vi "ChannelAutomatorR_Whole.vi"() -> ()   [LabVIEW 2024]
uses:
  E:/CodeProjects/DEMPbot/ChannelAutomatorR2/PumpAdapter.exe
  PumpAdapter.exe
  <vilib>/Analysis/baseanly.llb/Mean (DBL).vi
  <vilib>/DAQmx/write.llb/DAQmx Write (Analog DBL 1Chan 1Samp).vi
  <vilib>/DAQmx/create/channels.llb/DAQmx Create Channel (AO-Voltage-Basic).vi
  <vilib>/DAQmx/create/channels.llb/DAQmx Create Channel (AI-Voltage-Basic).vi
  <vilib>/DAQmx/miscellaneous.llb/DAQmx Fill In Error Info.vi
  <vilib>/DAQmx/configure/timing.llb/DAQmx Timing (Sample Clock).vi
  <vilib>/Analysis/NI_AALBase.lvlib
panel:
  in  "Run Experiment":bool
  out "Pull":string
  out "LastTDMS":refnum<k34>
  out "ChannelHistory":refnum<k24>
  out "Array":dbl[](array[numeric])
  out "Stats":string[][](table)
  out "History":cluster{dbl[], dbl[]}[](graph)
  out "Pump":refnum<k24>
  out "First Time":i64
  out "LastPoint":i64
  out "biasChannel":refnum<k21>
  out "HistoryArray":T1(array[cluster])
  out "MeasureMode":enum32{"RT Monitor", "IV Monitor"}(ring)
  out "error out 4":errorcluster
  out "fileCreateTime":timestamp
  out "error out 2":errorcluster
  in  "Tab Control 2":T2(tab)
  out "Channel 4":waveform(dbl)[](graph)
  out "Channel 3":waveform(dbl)[](graph)
  out "Channel 2":waveform(dbl)[](graph)
  out "Channel 1":waveform(dbl)[](graph)
  out "XY Graph":cluster{"Y":dbl[], "Y":dbl[]}[](graph)
  out "XY Graph 2":cluster{"Y":dbl[], "Y":dbl[]}[](graph)
  out "XY Graph 3":cluster{"Y":dbl[], "Y":dbl[]}[](graph)
  out "XY Graph 4":cluster{"Y":dbl[], "Y":dbl[]}[](graph)
  in  "Experiment":string[][](table)=[["Air", "", "Air", "0", "", "", "", "", "1", "200", "5", "IV Curve", "", ""], ["Air", "", "Air", "0", "", "", "", "", "5", "200", "5", "", "", ""], ["", "pushonly", "Water", "1800", "200", "", "", "", "", "", "", "", "", ""], ["TimEtch", "pushonly", "Waste", "500", "200", "", "", "", "", "50", "", "RT Start", "", ""], ["TE_Rinse", "", "Water", "3000", "200", "", "", "", "", "", "", " ", "", ""], ["", "", "", "0", "", "", "", "", "", "50", "", "RT End", "", ""], ["TE_Rinse", "", " ", "0", "", "", "", "", "5", "200", "5", "IV Curve", "", ""], ["MPA", "pullmore", "MPA", "300", "200", "", "1000", "", "", "", "", " ", "", ""], ["", "", "Air", "100", "200", "", "", "", "", "50", "", "RT Start", "", ""], ["MPA", "", "Water", "1600", "100", "", "", "", "", "", "", "", "", ""], ["", "", "MPA", "0", "", "", "", "", "0", "50", "", "RT End", "", ""], ["", "", "MPA", "0", "", "", "", "", "360", "100", "", "Burst", "60", "1"], ["MPA Rinse", "", "Water", "3000", "100", "", "", "", "60", "100", "", "", "", ""], ["MPA Rinse", "", "MPARinse", "0", "", "", "", "", "5", "100", "5", "IV Curve", "", ""], ["", "", "", "", "", "", "", "", "", "", "", "", "", ""], ["", "", "", "", "", "", "", "", "", "", "", "", "", ""], ["", "", "", "", "", "", "", "", "", "", "", "", "", ""], ["", "", "", "", "", "", "", "", "", "", "", "", "", ""], ["", "", "", "", "", "", "", "", "", "", "", "", "", ""], ["", "", "", "", "", "", "", "", "", "", "", "", "", ""], ["", "", "", "", "", "", "", "", "", "", "", "", "", ""], ["", "", "", "", "", "", "", "", "", "", "", "", "", ""]]
  out "output path":path
  out "FilenameValid":bool
  out "ParameterNames":string[](array[string])=["Wafer", "Notes", "Experiment Name", "Buffer", "Bias Voltage", "Reference Electrode", "Chip", "Analyte"]
  out "ParameterValues":string[](array[string])
  out "RT Monitoring 2":bool
  out "error out":errorcluster
  out "StopProgram":bool
  out "FileOpen":bool
  out "tdms file out":refnum<k34>
  in  "Tab Control":enum32{"Data View", "Automation", "Settings"}(tab)
  in  "Current Step":dbl
  in  "TraceTime":dbl=30.0
  in  "IV Monitoring":bool
  in  "RT Monitoring":bool
  out "Recording":bool
  in  "Record":bool
  in  "Reference Voltage (mV)":string="100"
  in  "Bias Voltage (mV)":string="100"
  in  "Experiment Name":string="asdf"
  in  "Wafer, Chip":string="asdf,a"
  in  "Notes":string
  in  "Buffer":string="asdf"
  in  "Analyte":string
  in  "DB48":bool
  in  "DB37":bool
  in  "Device Banks":bool
  in  "DB26":bool
  in  "Channels":string="N2,N6,E2,E6,S2,S6,W2,W6"
  out "Warnings":string="Wrong number of Channel Names!"
  out "Monitoring":bool
  out "frequency":dbl=20.0
  out "Running Experiment":bool
  in  "LoadPort":bool
  in  "Port To Clean":string="MPA"
  in  "CleanPort":bool
  in  "SyringeVolume":dbl=1000.0
  in  "CleanAll":bool
  in  "MPA Load":bool
  in  "PrimeWater":bool
  in  "TimeEtch Back":bool
  in  "ClearInput":bool
  in  "Clear Waste":bool
  in  "Dead Volume":dbl=3000.0
  in  "DataDirectory":path=path "C:/DempBot_Data"
  in  "Sampling Rate:":dbl=5000.0
  in  "Recorded Channels":i32=8
  in  "No. of Samples / Loop":i64=1000
  in  "Gain (V/nA)":dbl=0.45
  in  "Bias channel":tag="Dev1/ao0"
  in  "anayteNames":string[](array[string])=["Water", "TimEtch", "Air", "Dispense", "Waste", "MPA", "Biotin", "SA"]
  in  "Channels 2":tag[](array[tag])=["Dev1/ai0", "Dev1/ai1", "Dev1/ai2", "Dev1/ai3", "Dev1/ai4", "Dev1/ai5", "Dev1/ai6", "Dev1/ai7"]
  in  "MaxSyringSpeed":dbl=1000.0
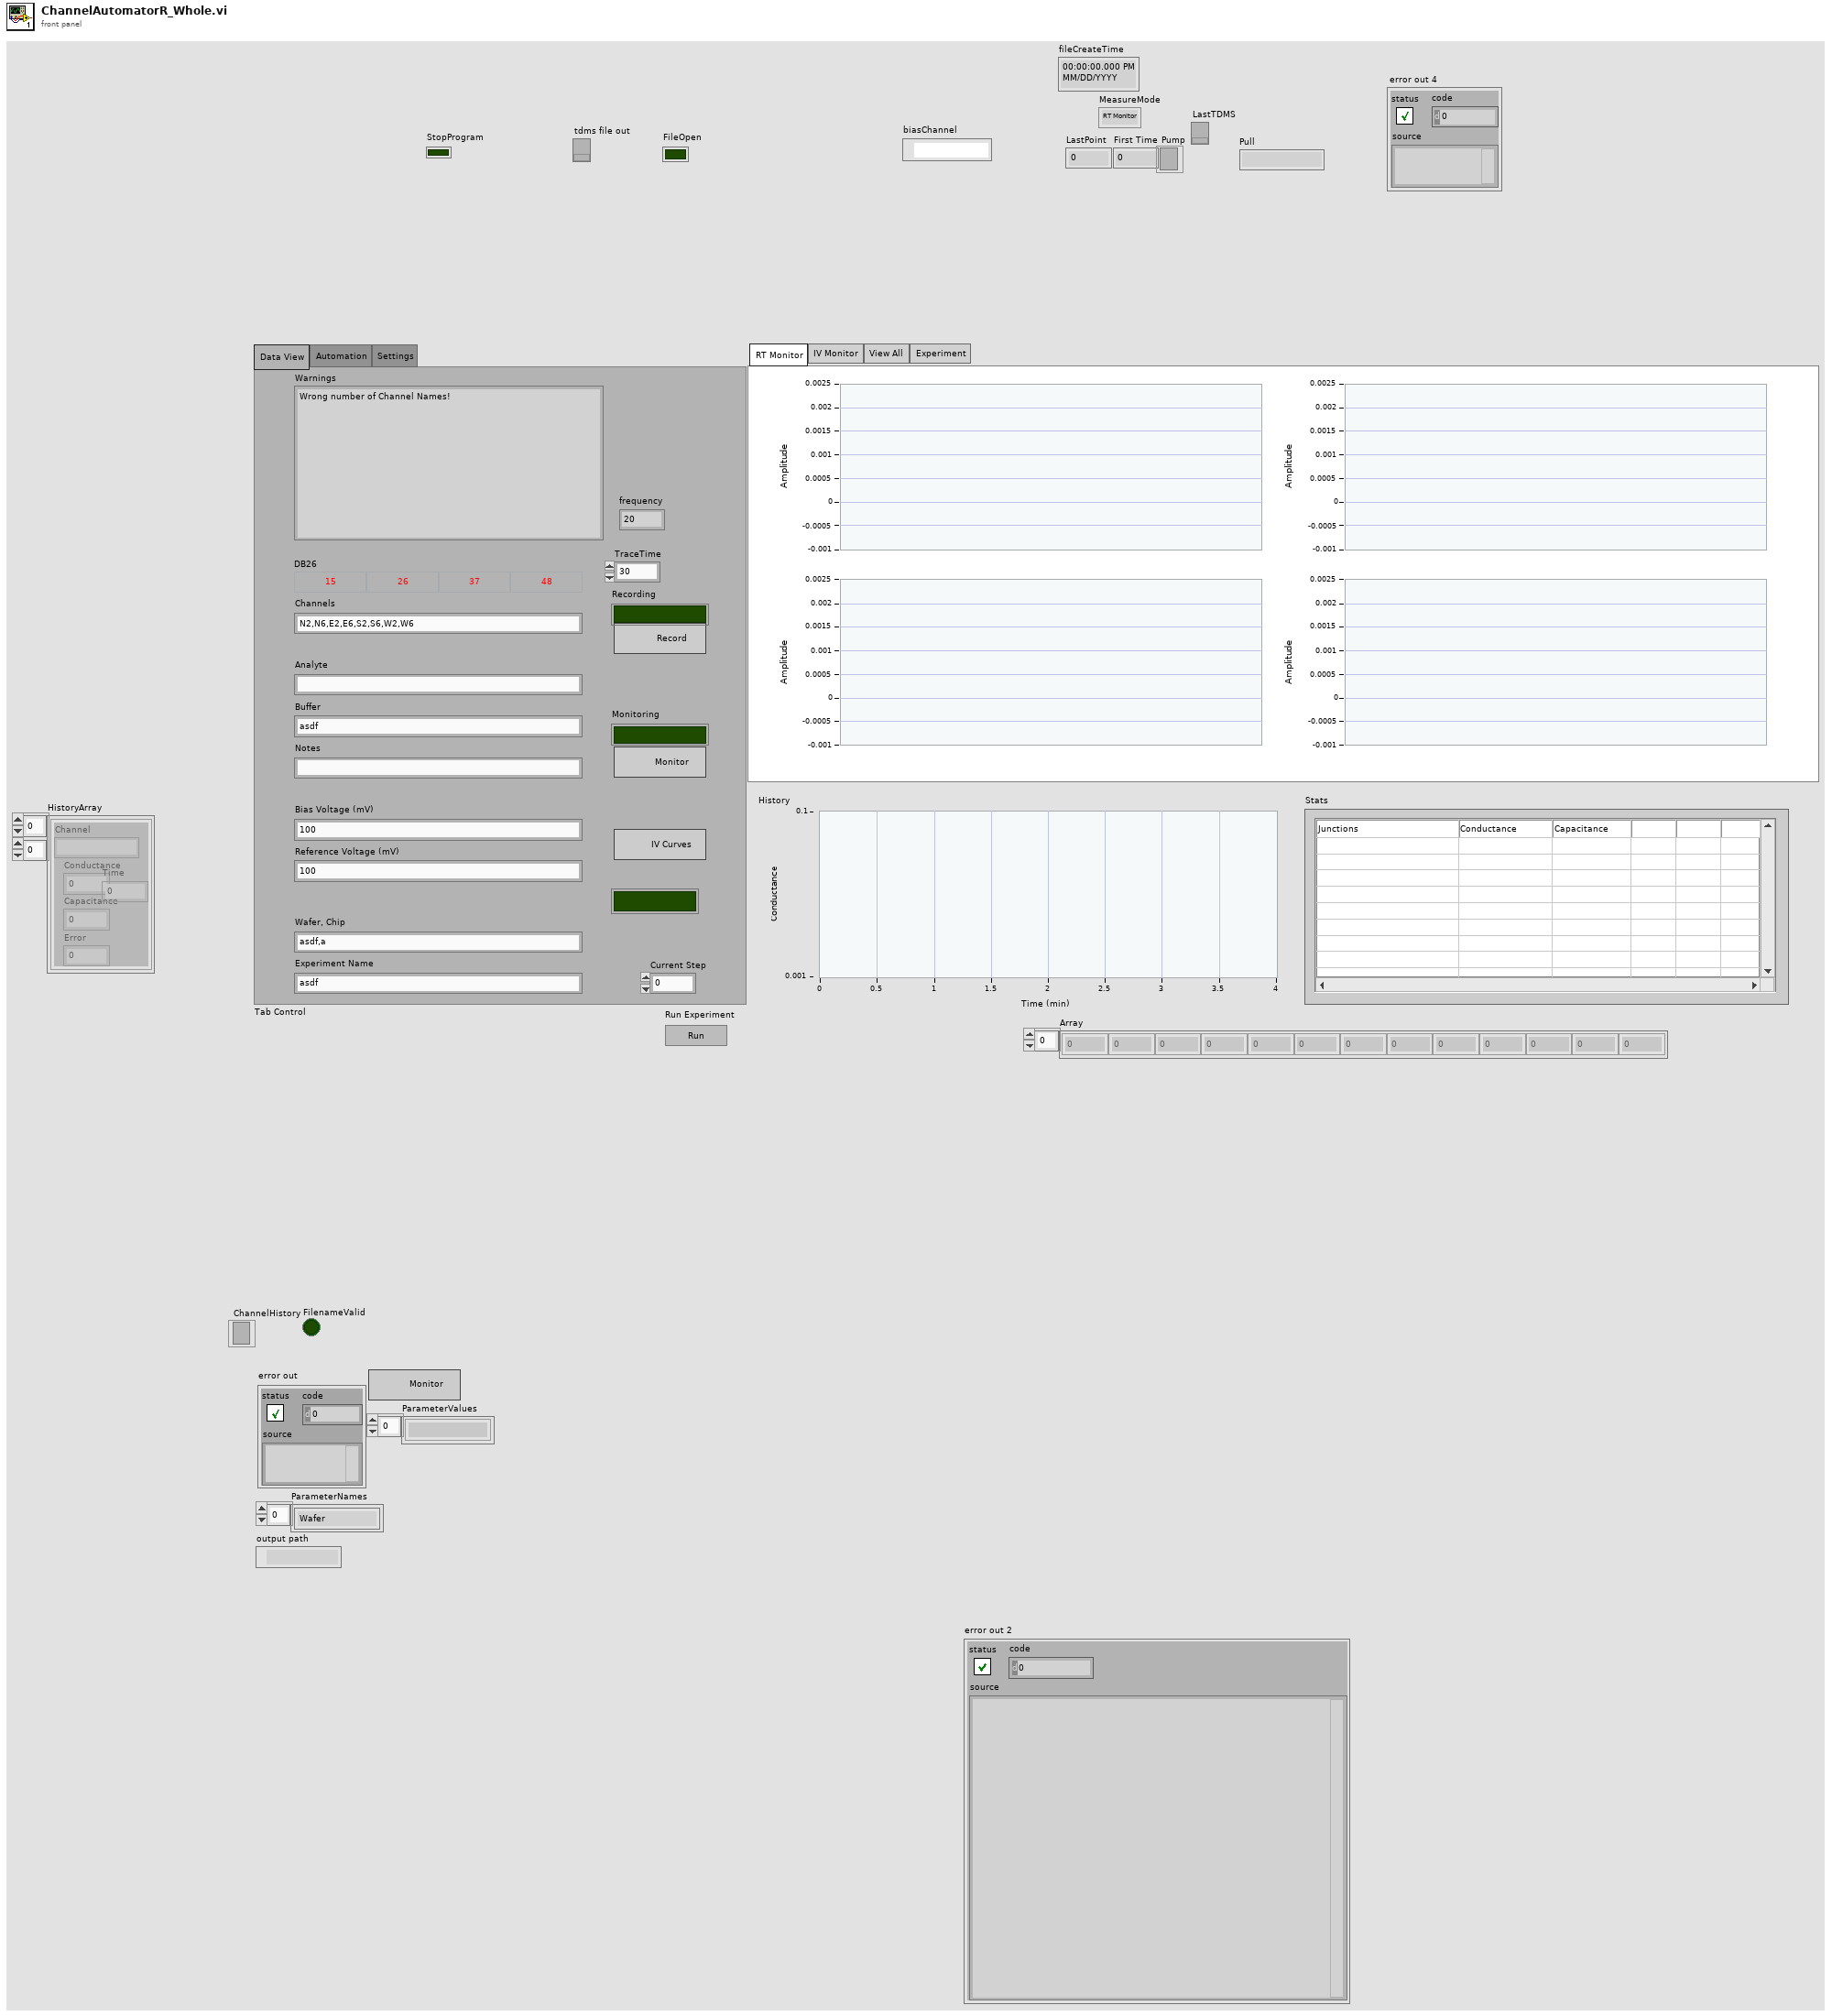
[diagram p1: front panel]
types:
  T1 = cluster{"Channel":string, "Conductance":dbl, "Capacitance":dbl, "Error":dbl, "Time":dbl}[][]
  T2 = enum32{"RT Monitor", "IV Monitor", "View All", "Experiment"}
  T3 = cluster{"Channel":string, "Conductance":dbl, "Capacitance":dbl, "Error":dbl}[][]
  T4 = typedef "MessageQueues.ctl" = cluster{"DelayTime":refnum<queue>, "DownSampled":refnum<queue>, "UserCommands":refnum<queue>, "InternalCommands":refnum<queue>, "CommandType":cluster{"Command":string}, "CommandAndPayload":cluster{"command":string, "machine":string, "payload":string}, "client handle out":T5, "PostData":string, "GetCommand":string, "Ack":string, "VoltageProgram":refnum<queue>, "ExperimentCommands":refnum<queue>, "DisplayCurrents":refnum<queue>, "MonitorCurrents":refnum<queue>, "FilePile":refnum<queue>}
  T5 = typedef "LabVIEWHTTPClient.lvlib/ClientHandle.ctl" = refnum<k1>
  T6 = enum16{"open", "open or create", "create or replace", "create", "open (read-only)"}
  T7 = cluster{"Waveforms":waveform(dbl)[], "file":refnum<k34>}[]
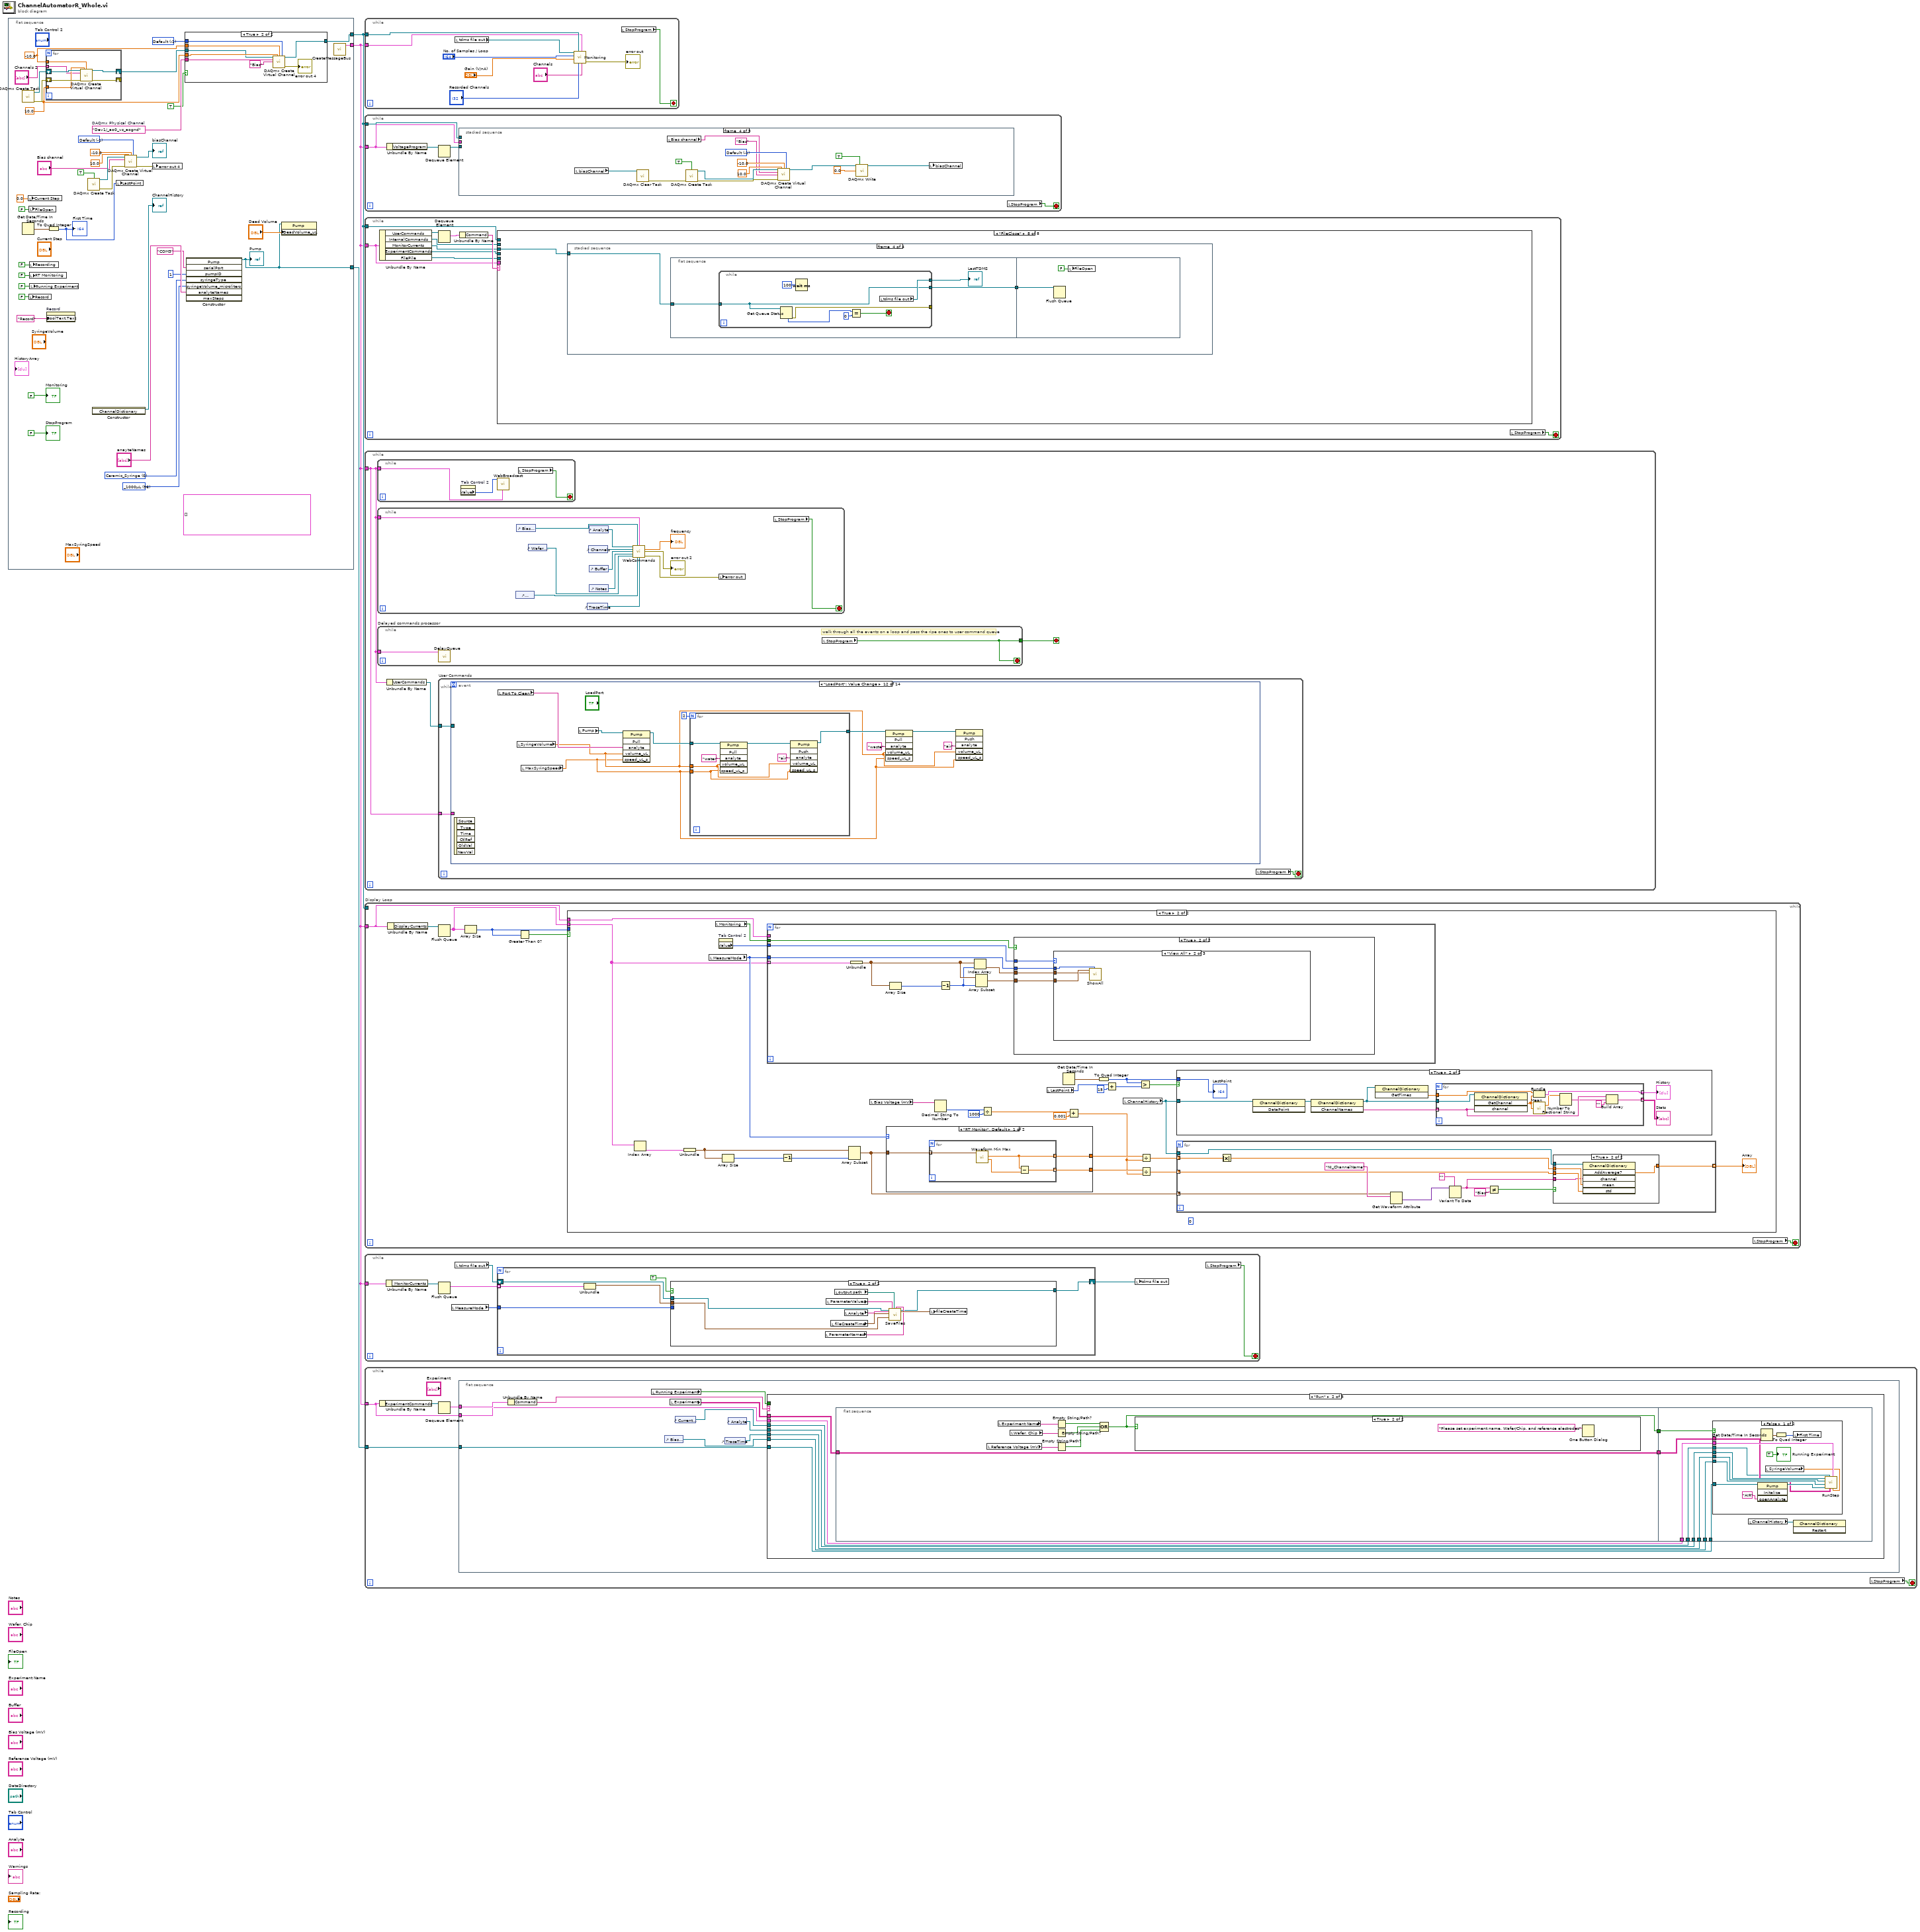
[diagram p0: block diagram]
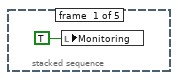
[diagram p7: hidden frame]
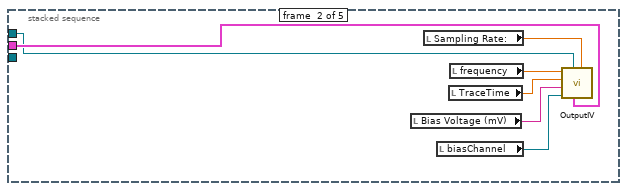
[diagram p8: hidden frame]
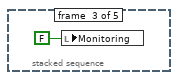
[diagram p9: hidden frame]
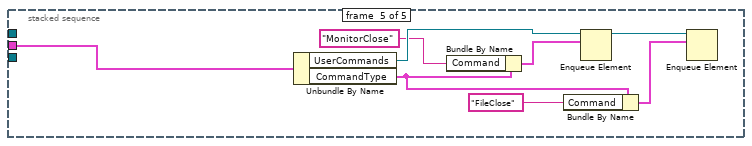
[diagram p10: hidden frame]
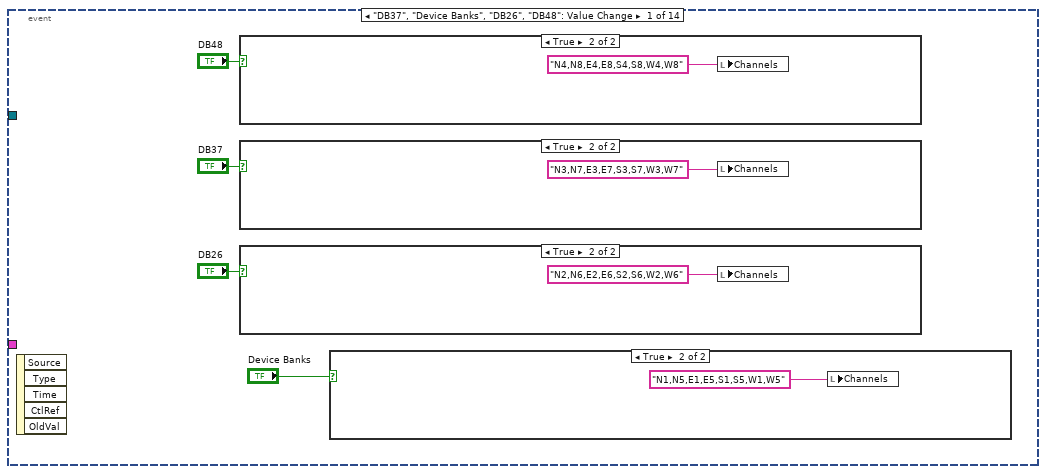
[diagram p11: hidden frame]
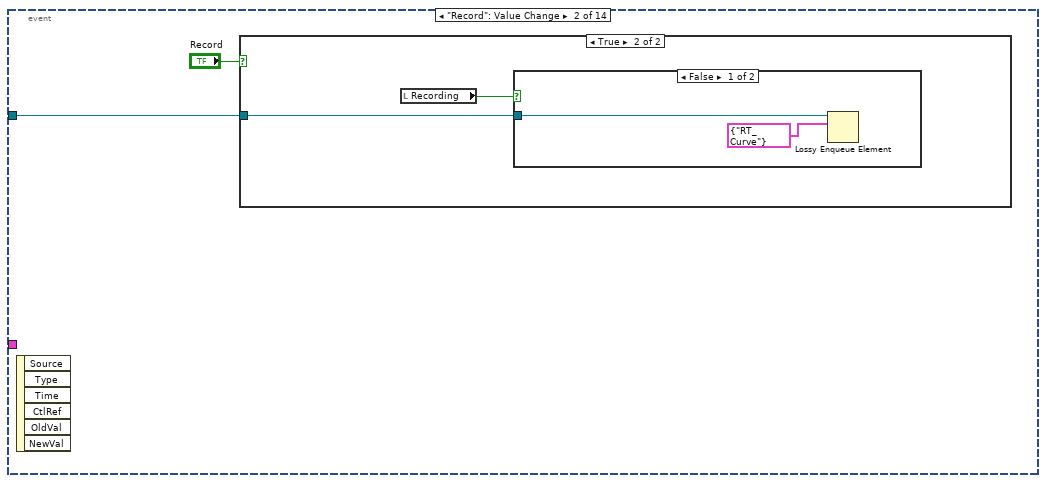
[diagram p16: hidden frame]
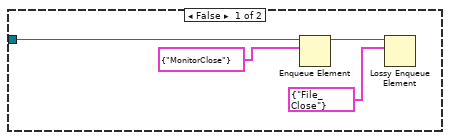
[diagram p17: hidden frame]
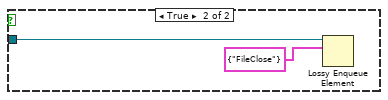
[diagram p18: hidden frame]
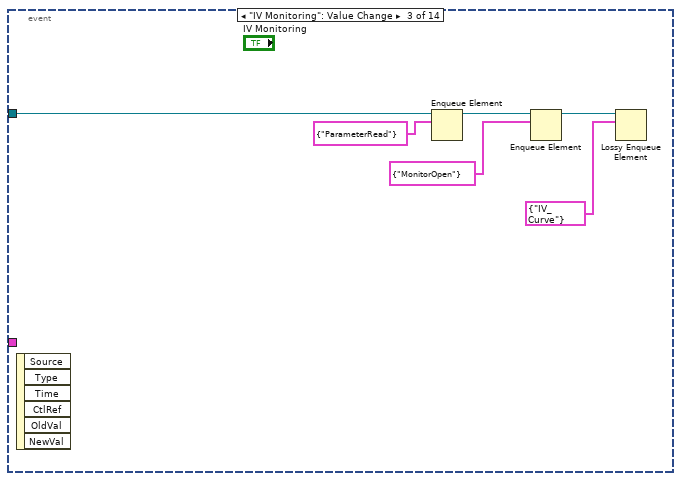
[diagram p19: hidden frame]
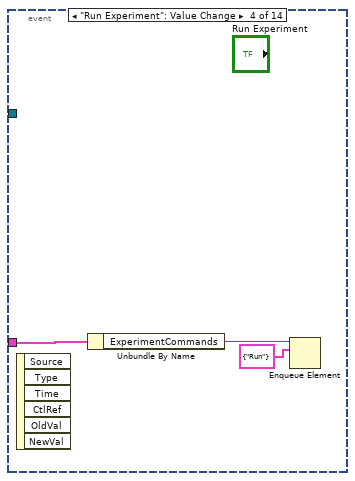
[diagram p20: hidden frame]
diagram:
  n1 = flat-sequence {
    tunnel: [w33] -> w2
    tunnel: [w28] -> w1
    tunnel: [w11] -> w3
    frame #0 {
      w8 = 0 items=["Ceramic_Syringe"=0, "Glass_Syringe"=2000, "Ceramic_Syringe_W_Wash"=2300, "Large_Glass_Syringe"=4000] ("syringeType")
      w9 = 96 items=["_250uL"=90, "_1250uL"=91, "_5000µL"=92, "_50µL"=93, "_100µL"=94, "_500µL"=95, "_1000µL"=96, "_2500µL"=97, "_12500µL"=98] ("syringeVolume_microliters")
      w23 = -1 items=["Default"=-1, "RSE"=10083, "Differential"=10106, "Pseudodifferential"=12529] ("output terminal configuration")
      (unwired) T3 []
      w31 = -1 items=["Default"=-1, "RSE"=10083, "NRSE"=10078, "Differential"=10106, "Pseudodifferential"=12529] ("input terminal configuration")
      w34 = tag "Dev1/_ao0_vs_aognd"  # DAQmx Physical Channel
      w30 = -10.0 ("minimum value")
      w29 = 10.0 ("maximum value")
      n2 = call <vilib>:"DAQmx Create Task.vi"() -> ("task out"=w42:refnum<k21>, "error out"=w41:errorcluster)  [unwired: 14 in]
      n3 = Get Date/Time In Seconds() -> (seconds since 1Jan1904=w13:timestamp)
      n4 = local write "Current Step"(0.0 ("Current Step")) -> ()
      n5 = local write "FileOpen"(FALSE ("FileOpen")) -> ()
      n6 = local write "Record"(FALSE ("Record")) -> ()
      n7 = local write "Recording"(FALSE ("Recording")) -> ()
      n8 = local write "RT Monitoring"(FALSE ("RT Monitoring")) -> ()
      n9 = local write "Running Experiment"(FALSE ("Running Experiment")) -> ()
      n10 = for {
        tunnel: w30 -> [w54]
        tunnel: w29 -> [w53]
        shift-right: [w58] -> w17
        shift-left: w42 -> [w56]
        shift-right: [w57] -> _
        shift-left: w41 -> [w55]
        tunnel: "Channels 2" -> [w52] mode=indexing
        n11 = call-poly <vilib>:"DAQmx Create Virtual Channel.vi"("task in"=w56, "maximum value"=w53, "minimum value"=w54, "physical channels"=w52, "error in"=w55) -> ("task out"=w58:refnum<k21>, "error out"=w57:errorcluster)  [unwired: 9 in]
      }
      n12 = property on="Record" class="Bool (strict)"("BoolText.Text"="Record" ("Boolean Text.Text")) -> ()  [unwired: 2 in, 2 out]
      n13 = To Quad Integer(1:w13) -> (0:w12:i64)
      "First Time" <- w12
      n14 = call <vilib>:"DAQmx Create Task.vi"("auto cleanup"=TRUE) -> ("task out"=w26:refnum<k21>, "error out"=w27:errorcluster)  [unwired: 13 in]
      n15 = constructor class="ChannelDictionary"() -> (reference out=→"ChannelHistory":refnum<k24>)  [unwired: 3 in, 2 out]
      n16 = local write "LastPoint"(w12) -> ()
      n17 = call-poly <vilib>:"DAQmx Create Virtual Channel.vi"("task in"=w26, "maximum value"=10.0, "minimum value"=-10.0, "output terminal configuration"=w23, "physical channels"="Bias channel", "error in"=w27) -> ("task out"=→"biasChannel":refnum<k21>, "error out"=w19:errorcluster)  [unwired: 8 in]
      n18 = local write "error out 4"(w19) -> ()
      n19 = case shown="True" TRUE {
        tunnel: w34 -> [_ w51]
        tunnel: [w43 w50] -> w33
        tunnel: w31 -> [_ w48]
        tunnel: w30 -> [_ w47]
        tunnel: w29 -> [_ w46]
        tunnel: w17 -> [w43 w44]
        frame False {
        }
        frame True {
          n20 = call-poly <vilib>:"DAQmx Create Virtual Channel.vi"("task in"=w44, "maximum value"=w46, "minimum value"=w47, "input terminal configuration"=w48, "physical channels"=w51, "name to assign"="Bias") -> ("task out"=w50:refnum<k21>, "error out"=→"error out 4":errorcluster)  [unwired: 8 in]
        }
      }
      n21 = constructor class="Pump"("serialPort"="COM3", "pumpID"=1, "syringeType"=w8, "syringeVolume_microliters"=w9, "analyteNames"="anayteNames") -> (reference out=w11:refnum<k24>)  [unwired: 4 in, 8 out]
      "Pump" <- w11
      n22 = property class="Pump"(reference=w11, "DeadVolume_uL"="Dead Volume") -> ()  [unwired: 1 in, 2 out]
      n23 = call "CreateMessageBus.vi"() -> ("MessageQueues"=w28:T4)  [unwired: 11 in]
      "StopProgram" <- FALSE ("StopProgram")
      "Monitoring" <- FALSE ("Monitoring")
    }
  }
  n24 = while {
    tunnel: w2 -> [w67]
    tunnel: w1 -> [w66]
    stop <- w60 stop-if-true
    n25 = local read "tdms file out"() -> (w59:refnum<k34>)
    n26 = call "Monitoring.vi"("Channels"="Channels", "MessageQueues"=w66, "Recorded Channels"="Recorded Channels", "task in"=w67, "Gain (V/nA)"="Gain (V/nA)", "No. of Samples / Loop"="No. of Samples / Loop", "tdms file out"=w59) -> ("error out"=→"error out":errorcluster)  [unwired: 4 in]
    n27 = local read "StopProgram"() -> (w60:bool)
  }
  n28 = while {
    tunnel: w1 -> [w71]
    tunnel: w2 -> [w70]
    stop <- w72 stop-if-true
    n29 = Unbundle By Name(w71) -> ("VoltageProgram"=w69:refnum<queue>)
    n30 = Dequeue Element(queue=w69) -> (queue out=w68:refnum<queue>)  [unwired: 2 in, 3 out]
    n31 = stacked-sequence {
      tunnel: w68 -> [_ _ _ _ _]
      tunnel: w71 -> [_ w77 _ _ w96]
      tunnel: w70 -> [_ w74 _ _ _]
      frame #0 {
        n32 = local write "Monitoring"(TRUE ("Monitoring")) -> ()
      }
      frame #1 {
        n33 = local read "Bias Voltage (mV)"() -> (w78:string)
        n34 = local read "Sampling Rate:"() -> (w75:dbl)
        n35 = local read "biasChannel"() -> (w76:refnum<k21>)
        n36 = local read "TraceTime"() -> (w80:dbl)
        n37 = local read "frequency"() -> (w79:dbl)
        n38 = call "OutputIV.vi"("Sampling Rate:"=w75, "MessageQueues"=w77, "MonitorTask"=w74, "BiasChannel"=w76, "Bias Voltage (mV)"=w78, "TraceTime"=w80, "frequency"=w79) -> ()  [unwired: 5 in]
      }
      frame #2 {
        n39 = local write "Monitoring"(FALSE ("Monitoring")) -> ()
      }
      frame #3 {
        w91 = -1 items=["Default"=-1, "RSE"=10083, "Differential"=10106, "Pseudodifferential"=12529] ("output terminal configuration")
        n40 = local read "biasChannel"() -> (w83:refnum<k21>)
        n41 = call <vilib>:"DAQmx Clear Task.vi"("task in"=w83) -> ("error out"=w82:errorcluster)  [unwired: 14 in]
        n42 = local read "Bias channel"() -> (w89:tag)
        n43 = call <vilib>:"DAQmx Create Task.vi"("auto cleanup"=TRUE, "error in"=w82) -> ("task out"=w94:refnum<k21>, "error out"=w95:errorcluster)  [unwired: 12 in]
        n44 = call-poly <vilib>:"DAQmx Create Virtual Channel.vi"("task in"=w94, "maximum value"=10.0, "minimum value"=-10.0, "output terminal configuration"=w91, "physical channels"=w89, "name to assign"="Bias", "error in"=w95) -> ("task out"=w86:refnum<k21>)  [unwired: 7 in, 1 out]
        n45 = call-poly <vilib>:"DAQmx Write.vi"("task/channels in"=w86, "auto start"=TRUE, "data"=0.0) -> ("task out"=w85:refnum<k21>)  [unwired: 10 in, 2 out]
        n46 = local write "biasChannel"(w85) -> ()
      }
      frame #4 {
        n47 = Unbundle By Name(w96) -> ("UserCommands"=w103:refnum<queue>, "CommandType"=w97:cluster{"Command":string})
        n48 = Bundle By Name(cluster=w97, "Command"="MonitorClose") -> (w102:cluster{"Command":string})
        n49 = Bundle By Name(cluster=w97, "Command"="FileClose") -> (w99:cluster{"Command":string})
        n50 = Enqueue Element(queue=w103, element=w102) -> (queue out=w100:refnum<queue>)  [unwired: 2 in, 2 out]
        n51 = Enqueue Element(queue=w100, element=w99) -> ()  [unwired: 2 in, 3 out]
      }
    }
    n52 = local read "StopProgram"() -> (w72:bool)
  }
  n53 = while {
    tunnel: w1 -> [w108]
    tunnel: w2 -> [w107]
    stop <- w113 stop-if-true
    n54 = Unbundle By Name(w108) -> ("UserCommands"=w110:refnum<queue>, "InternalCommands"=w109:refnum<queue>, "MonitorCurrents"=w106:refnum<queue>, "ExperimentCommands"=w105:refnum<queue>, "FilePile"=w104:refnum<queue>)
    n55 = Dequeue Element(queue=w110) -> (element=w112:cluster{"Command":string})  [unwired: 2 in, 3 out]
    n56 = Unbundle By Name(w112) -> ("Command"=w111:string)
    n57 = case shown="\"FileClose\"" w111 {
      tunnel: w107 -> [w115 w166 _ _ _ w262 _ _]
      tunnel: w109 -> [w117 w165 w188 _ _ w261 _ _]
      tunnel: w108 -> [w116 _ w189 _ _ _ _ _]
      tunnel: w106 -> [_ _ _ _ _ w259 _ w277]
      tunnel: w105 -> [_ _ _ _ _ w258 _ _]
      tunnel: w104 -> [w114 _ w187 _ _ _ _ _]
      frame "RT_Curve" {
        n58 = local read "FilenameValid"() -> (w118:bool)
        n59 = case shown="True" w118 {
          tunnel: w117 -> [w119 _]
          tunnel: w116 -> [_ w124]
          tunnel: w115 -> [_ w125]
          tunnel: w114 -> [_ w123]
          frame False {
            n60 = property on="Record" class="Bool (strict)"("BoolText.Text"="Record" ("Boolean Text.Text")) -> ()  [unwired: 2 in, 2 out]
            n61 = Lossy Enqueue Element(queue=w119, element=cluster{"Command":string} {"Command"="MonitorClose"}) -> ()  [unwired: 1 in, 4 out]
            n62 = local write "Warnings"("Wafer, Chip and Analyte must be filled" ("Warnings")) -> ()
          }
          frame True {
            n63 = stacked-sequence {
              tunnel: w125 -> [_ w163]
              tunnel: w124 -> [_ w162]
              tunnel: w123 -> [w129 _]
              frame #0 {
                w133 = enum32{"RT Monitor", "IV Monitor"}."RT Monitor" ("Tab Control 2")
                n64 = local write "FileOpen"(TRUE ("FileOpen")) -> ()
                n65 = local write "Recording"(TRUE ("Recording")) -> ()
                n66 = local write "Monitoring"(TRUE ("Monitoring")) -> ()
                n67 = local read "output path"() -> (w143:path)
                n68 = property on="Record" class="Bool (strict)"("BoolText.Text"="Stop" ("Boolean Text.Text")) -> ()  [unwired: 2 in, 2 out]
                n69 = call <vilib>:"Check if File or Folder Exists.vi"("path"=w143) -> ("file or folder exists?"=w136:bool, "dup path"=w140:path)  [unwired: 8 in, 1 out]
                n70 = Get Date/Time In Seconds() -> (seconds since 1Jan1904=w147:timestamp)
                n71 = case shown="False" w136 {
                  tunnel: w140 -> [w156 w157]
                  tunnel: [w155 w157] -> w138
                  frame False {
                    n72 = Create Folder(path (use dialog)=w156) -> (created path=w155:path)  [unwired: 2 in, 2 out]
                  }
                  frame True {
                  }
                }
                n73 = local write "fileCreateTime"(w147) -> ()
                n74 = local read "Analyte"() -> (w148:string)
                n75 = Format Date/Time String(time format string (%c)="%y%m%d_%H%M%S_", seconds (now)=w147) -> (date/time string=w149:string)  [unwired: 1 in]
                n76 = Concatenate Strings(w149, w148, "RT.tdms" ("string")) -> (w150:string)
                n77 = local read "ParameterNames"() -> (w141:string[])
                n78 = Build Path(base path=w138, name or relative path=w150) -> (appended path=w139:path)
                n79 = local read "ParameterValues"() -> (w142:string[])
                n80 = property on="Tab Control 2" class="TabCtl (strict)"("Value"=w133) -> ()  [unwired: 2 in, 2 out]
                n81 = Format Into String(w133) -> (resulting string=w145:string)  [unwired: 3 in, 1 out]
                n82 = Build Array (concatenate)(w141, "Mode") -> (w146:string[])
                n83 = Build Array (concatenate)(w142, w145) -> (w144:string[])
                n84 = TDMS Open(5:FALSE ("create index file? (T)"), 10:T6."create" ("operation (0:open)"), 11:w139) -> (3:w137:refnum<k34>)  [unwired: 4 in, 1 out]
                n85 = TDMS Set Properties(5:w144, 7:w146, 11:w137) -> (3:w126:refnum<k34>)  [unwired: 3 in, 3 out]
                "tdms file out" <- w126
                n86 = Bundle By Name(cluster=cluster{"file":refnum<k34>} {"file"=refnum} ("element"), "file"=w126) -> (w127:cluster{"file":refnum<k34>})
                n87 = Enqueue Element(queue=w129, element=w127) -> ()  [unwired: 2 in, 3 out]
                "MeasureMode" <- w133
              }
              frame #1 {
                n88 = local read "Bias Voltage (mV)"() -> (w160:string)
                n89 = local read "Sampling Rate:"() -> (w159:dbl)
                n90 = local read "biasChannel"() -> (w158:refnum<k21>)
                n91 = call "OutputRT.vi"("Bias in"=w158, "Monitor Task"=w163, "rate"=w159, "MessageQueues"=w162, "Bias Voltage (mV)"=w160, "TraceTime"="TraceTime") -> ()  [unwired: 6 in]
              }
            }
          }
        }
      }
      frame "MonitorOpen" {
        n92 = local read "biasChannel"() -> (w164:refnum<k21>)
        n93 = stacked-sequence {
          seq-local: [w171 _ _] -> [_ w174 _]
          seq-local: [w170 _ _] -> [_ w176 _]
          seq-local: [_ w175 _] -> [_ _ _]
          tunnel: w166 -> [w173 _ _]
          tunnel: w164 -> [w169 _ _]
          tunnel: [w168 _ _] -> _
          tunnel: w165 -> [_ _ w185]
          frame #0 {
            n94 = local write "FileOpen"(FALSE ("FileOpen")) -> ()
            n95 = local write "Monitoring"(TRUE ("Monitoring")) -> ()
            n96 = call <vilib>:"DAQmx Stop Task.vi"("task/channels in"=w173) -> ("task out"=w171:refnum<k21>)  [unwired: 13 in, 1 out]
            n97 = call <vilib>:"DAQmx Stop Task.vi"("task/channels in"=w169) -> ("task out"=w170:refnum<k21>, "error out"=w168:errorcluster)  [unwired: 13 in]
          }
          frame #1 {
            w184 = 10123 items=["Finite Samples"=10178, "Continuous Samples"=10123, "Hardware Timed Single Point"=12522] ("sample mode")
            n98 = local read "Bias Voltage (mV)"() -> (w177:string)
            n99 = Decimal String To Number(string=w177, default (0L)=0.0) -> (number=w180:dbl)  [unwired: 1 in, 1 out]
            n100 = Divide(x=w180, y=1000) -> (x/y=w179:dbl)
            n101 = call-poly <vilib>:"DAQmx Write.vi"("task/channels in"=w176, "auto start"=TRUE, "data"=w179) -> ()  [unwired: 10 in, 3 out]
            n102 = local read "Sampling Rate:"() -> (w183:dbl)
            n103 = call-poly <vilib>:"DAQmx Timing.vi"("task/channels in"=w174, "sample mode"=w184, "rate"=w183) -> ("task out"=w175:refnum<k21>)  [unwired: 11 in, 1 out]
          }
          frame #2 {
            n104 = Lossy Enqueue Element(queue=w185, element=cluster{"Command":string} {"Command"="Monitor"}) -> ()  [unwired: 1 in, 4 out]
          }
        }
      }
      frame "IV_Curve" {
        n105 = local read "FilenameValid"() -> (w190:bool)
        n106 = case shown="True" w190 {
          tunnel: w189 -> [_ w199]
          tunnel: w188 -> [_ w197]
          tunnel: w187 -> [_ w196]
          frame False {
            n107 = Obtain Queue(name (unnamed)="InternalCommands", element data type=cluster{"Command":string} {"Command"=""}, create if not found? (T)=FALSE) -> (queue out=w191:refnum<queue>)  [unwired: 2 in, 2 out]
            n108 = Lossy Enqueue Element(queue=w191, element=cluster{"Command":string} {"Command"="MonitorClose"}) -> ()  [unwired: 1 in, 4 out]
          }
          frame True {
            n109 = Unbundle By Name(w199) -> ("VoltageProgram"=w198:refnum<queue>)
            n110 = stacked-sequence {
              seq-local: [w200 _ _] -> [_ w226 _]
              tunnel: w198 -> [_ _ w233]
              tunnel: w197 -> [_ _ w231]
              tunnel: w196 -> [_ w225 _]
              frame #0 {
                w206 = enum32{"RT Monitor", "IV Monitor"}."IV Monitor" ("Tab Control 2")
                n111 = local read "output path"() -> (w212:path)
                n112 = call <vilib>:"Check if File or Folder Exists.vi"("path"=w212) -> ("file or folder exists?"=w207:bool, "dup path"=w210:path)  [unwired: 8 in, 1 out]
                n113 = Get Date/Time In Seconds() -> (seconds since 1Jan1904=w220:timestamp)
                "fileCreateTime" <- w220
                n114 = case shown="False" w207 {
                  tunnel: w210 -> [w223 w224]
                  tunnel: [w222 w224] -> w209
                  frame False {
                    n115 = Create Folder(path (use dialog)=w223) -> (created path=w222:path)  [unwired: 2 in, 2 out]
                  }
                  frame True {
                  }
                }
                n116 = local read "Analyte"() -> (w214:string)
                n117 = Format Date/Time String(time format string (%c)="%y%m%d_%H%M%S_", seconds (now)=w220) -> (date/time string=w213:string)  [unwired: 1 in]
                n118 = Concatenate Strings(w213, w214, "IV.tdms" ("string")) -> (w215:string)
                n119 = local read "ParameterNames"() -> (w216:string[])
                n120 = Build Path(base path=w209, name or relative path=w215) -> (appended path=w211:path)
                n121 = local read "ParameterValues"() -> (w217:string[])
                n122 = property on="Tab Control 2" class="TabCtl (strict)"("Value"=w206) -> ()  [unwired: 2 in, 2 out]
                n123 = local write "MeasureMode"(w206) -> ()
                n124 = Format Into String(w206) -> (resulting string=w221:string)  [unwired: 3 in, 1 out]
                n125 = Build Array (concatenate)(w216, "mode") -> (w219:string[])
                n126 = Build Array (concatenate)(w217, w221) -> (w218:string[])
                n127 = TDMS Open(5:FALSE ("create index file? (T)"), 10:T6."create" ("operation (0:open)"), 11:w211) -> (3:w208:refnum<k34>)  [unwired: 4 in, 1 out]
                n128 = TDMS Set Properties(5:w218, 7:w219, 11:w208) -> (3:w200:refnum<k34>)  [unwired: 3 in, 3 out]
              }
              frame #1 {
                n129 = local write "FileOpen"(TRUE ("FileOpen")) -> ()
                n130 = local write "tdms file out"(w226) -> ()
                n131 = Bundle By Name(cluster=cluster{"file":refnum<k34>} {"file"=refnum} ("element"), "file"=w226) -> (w227:cluster{"file":refnum<k34>})
                n132 = Enqueue Element(queue=w225, element=w227) -> ()  [unwired: 2 in, 3 out]
              }
              frame #2 {
                n133 = Enqueue Element(queue=w231, element=cluster{"Command":string} {"Command"="Monitor"}) -> ()  [unwired: 2 in, 3 out]
                n134 = Enqueue Element(queue=w233, element=cluster{"Command":string, "Time":i32} {"Command"="IV", "Time"=0}) -> ()  [unwired: 2 in, 3 out]
              }
            }
          }
        }
      }
      frame Default {
      }
      frame "ParameterRead" {
        w246 = "" ("y")
        n135 = local read "Wafer, Chip"() -> (w244:string)
        n136 = local read "Analyte"() -> (w240:string)
        n137 = Not Equal?(x=w244, y=w246) -> (x != y?=w235:bool)
        n138 = Not Equal?(x=w240, y=w246) -> (x != y?=w237:bool)
        n139 = call <vilib>:"Delimited String to 1D String Array.vi"("delimiter"="," ("search string/char (-)"), "delimited string"=w244) -> ("string array"=w242:string[])  [unwired: 9 in]
        n140 = local read "Reference Voltage (mV)"() -> (w248:string)
        n141 = local read "Experiment Name"() -> (w251:string)
        n142 = local read "Bias Voltage (mV)"() -> (w249:string)
        n143 = local read "DataDirectory"() -> (w247:path)
        n144 = Or(x=w237, y=w235) -> (x .or. y?=→"FilenameValid":bool)
        n145 = Index Array(array=w242) -> (element #1=w241:string, element #2=w239:string)  [unwired: 2 in]
        n146 = Build Path(base path=w247, name or relative path=w241) -> (appended path=w238:path)
        n147 = local read "Notes"() -> (w252:string)
        n148 = local read "Buffer"() -> (w250:string)
        n149 = Build Array(w241, w252, w251, w250, w249, w248, w239, w240) -> (→"ParameterValues":string[])
        n150 = Build Path(base path=w238, name or relative path=w239) -> (appended path=→"output path":path)
        "ParameterNames" <- string[] ["Wafer", "Notes", "Experiment Name", "Buffer", "Bias Voltage", "Reference Electrode", "Chip", "Analyte"]
      }
      frame "MonitorClose" {
        n151 = local write "Monitoring"(FALSE ("Monitoring")) -> ()
        n152 = local read "biasChannel"() -> (w260:refnum<k21>)
        n153 = Bundle By Name("Y"=dbl[] []) -> (w257:waveform(dbl))  [unwired: 1 in]
        n154 = stacked-sequence {
          seq-local: [w264 _ _] -> [_ w269 _]
          seq-local: [_ w268 _] -> [_ _ w275]
          seq-local: [_ w266 _] -> [_ _ w274]
          tunnel: w262 -> [w265 _ _]
          tunnel: w260 -> [w264 _ _]
          tunnel: w261 -> [_ w270 _]
          tunnel: w259 -> [_ w267 _]
          tunnel: [_ _ w275] -> _
          tunnel: w258 -> [_ _ w273]
          frame #0 {
            n155 = call <vilib>:"DAQmx Stop Task.vi"("task/channels in"=w265) -> ()  [unwired: 13 in, 2 out]
          }
          frame #1 {
            n156 = Lossy Enqueue Element(queue=w270, element=cluster{"Command":string} {"Command"="Close"}) -> ()  [unwired: 1 in, 4 out]
            n157 = Flush Queue(queue=w267) -> (queue out=w266:refnum<queue>)  [unwired: 1 in, 2 out]
            n158 = call <vilib>:"DAQmx Stop Task.vi"("task/channels in"=w269) -> ("error out"=w268:errorcluster)  [unwired: 13 in, 1 out]
          }
          frame #2 {
            n159 = Enqueue Element(queue=w273, element=cluster{"Command":string} {"Command"="Step"}) -> ()  [unwired: 2 in, 3 out]
            n160 = Flush Queue(queue=w274) -> ()  [unwired: 1 in, 3 out]
          }
        }
        n161 = Build Array(w257) -> (w256:waveform(dbl)[])
        n162 = Build Array(w256) -> (w254:waveform(dbl)[][])
        n163 = property on="Channel 1" class="WFChart (strict)"("History Data"=w254) -> ()  [unwired: 2 in, 2 out]
        n164 = property on="Channel 2" class="WFChart (strict)"("History Data"=w254) -> ()  [unwired: 2 in, 2 out]
        n165 = property on="Channel 3" class="WFChart (strict)"("History Data"=w254) -> ()  [unwired: 2 in, 2 out]
        n166 = property on="Channel 4" class="WFChart (strict)"("History Data"=w254) -> ()  [unwired: 2 in, 2 out]
      }
      frame "DisplayClose" {
        n167 = local write "Monitoring"(FALSE ("Monitoring")) -> ()
      }
      frame "FileClose" {
        n168 = stacked-sequence {
          tunnel: w277 -> [_ w282 _ w285]
          frame #0 {
            w278 = FALSE ("RT Monitoring")
            n169 = property on="Record" class="Bool (strict)"("Value"=FALSE ("Record")) -> ()  [unwired: 2 in, 2 out]
            n170 = property on="RT Monitoring" class="Bool (strict)"("Value"=w278) -> ()  [unwired: 2 in, 2 out]
            n171 = property on="IV Monitoring" class="Bool (strict)"("Value"=w278) -> ()  [unwired: 2 in, 2 out]
            n172 = property on="Record" class="Bool (strict)"("BoolText.Text"="Record" ("Boolean Text.Text")) -> ()  [unwired: 2 in, 2 out]
            n173 = local write "Warnings"("File has been saved" ("Warnings")) -> ()
          }
          frame #1 {
            n174 = Flush Queue(queue=w282) -> ()  [unwired: 1 in, 3 out]
          }
          frame #2 {
            n175 = local write "Recording"(FALSE ("Recording")) -> ()
          }
          frame #3 {
            n176 = flat-sequence {
              tunnel: w285 -> [w288]
              tunnel: [w286] -> w284
              tunnel: w284 -> [w296]
              frame #0 {
                n177 = while {
                  tunnel: w288 -> [w289]
                  tunnel: [w291] -> _
                  tunnel: [w290] -> w287
                  tunnel: [w289] -> w286
                  stop <- w293 stop-if-true
                  n178 = Get Queue Status(queue=w289) -> (error out=w291:errorcluster, # elements in queue=w295:i32)  [unwired: 2 in, 6 out]
                  n179 = Wait (ms)(milliseconds to wait=u32 100) -> ()  [unwired: 1 out]
                  n180 = Equal?(x=w295, y=0) -> (x = y?=w293:bool)
                  n181 = local read "tdms file out"() -> (w290:refnum<k34>)
                }
                "LastTDMS" <- w287
              }
              frame #1 {
                n182 = Flush Queue(queue=w296) -> ()  [unwired: 1 in, 3 out]
                n183 = local write "FileOpen"(FALSE ("FileOpen")) -> ()
              }
            }
          }
        }
      }
    }
    n184 = local read "StopProgram"() -> (w113:bool)
  }
  n185 = while {
    tunnel: w1 -> [w298]
    stop <- w300 stop-if-true
    n186 = while {
      tunnel: w298 -> [w498]
      stop <- w500 stop-if-true
      n187 = property on="Tab Control 2" class="TabCtl (strict)"() -> ("Value"=w499:T2)  [unwired: 2 in, 2 out]
      n188 = call "WebBroadcast.vi"("MessageQueues"=w498, "Measure Mode"=w499) -> ()  [unwired: 10 in]
      n189 = local read "StopProgram"() -> (w500:bool)
    }
    n190 = while {
      tunnel: w298 -> [w501]
      stop <- w513 stop-if-true
      n191 = control-ref of="Experiment Name"() -> (w505:refnum<vi>)
      n192 = control-ref of="Bias Voltage (mV)"() -> (w510:refnum<vi>)
      n193 = control-ref of="Wafer, Chip"() -> (w506:refnum<vi>)
      n194 = control-ref of="TraceTime"() -> (w504:refnum<vi>)
      n195 = control-ref of="Channels"() -> (w509:refnum<vi>)
      n196 = control-ref of="Analyte"() -> (w511:refnum<vi>)
      n197 = control-ref of="Buffer"() -> (w508:refnum<vi>)
      n198 = control-ref of="Notes"() -> (w507:refnum<vi>)
      n199 = call "WebCommands.vi"("Analyte"=w511, "Bias"=w510, "MessageQueues"=w501, "channels"=w509, "buffer"=w508, "notes"=w507, "waferChip"=w506, "experiment"=w505, "reference 8"=w504) -> ("frequency"=→"frequency":dbl, "error out 2"=→"error out 2":errorcluster, "error out"=w512:errorcluster)  [unwired: 4 in]
      n200 = local write "error out"(w512) -> ()
      n201 = local read "StopProgram"() -> (w513:bool)
    }
    n202 = while "Delayed commands processor" {
      tunnel: w298 -> [w497]
      tunnel: [w496] -> w300
      stop <- w496 stop-if-true
      # "walk through all the events on a loop and pass the ripe ones to user command queue"
      n203 = call "DelayQueue.vi"("MessageQueues"=w497) -> ()  [unwired: 11 in]
      n204 = local read "StopProgram"() -> (w496:bool)
    }
    n205 = Unbundle By Name(w298) -> ("UserCommands"=w299:refnum<queue>)
    n206 = while "User Commands" {
      tunnel: w299 -> [w302]
      tunnel: w298 -> [w301]
      stop <- w303 stop-if-true
      n207 = event shown="[11] \"LoadPort\": Value Change" {
        selector: _ -> [_ _ _ _ _ _ _ _ _ _ _ _ _ _]
        dyn-events: _ -> [_ _ _ _ _ _ _ _ _ _ _ _ _ _]
        timeout: _ -> [_ _ _ _ _ _ _ _ _ _ _ _ _ _]
        tunnel: w302 -> [_ w312 w324 _ w333 _ _ _ _ _ _ _ _ w494]
        tunnel: w301 -> [_ _ _ w332 _ _ _ _ _ _ _ _ _ _]
        event "DB37", "Device Banks", "DB26", "DB48": Value Change {
          n208 = event-data() -> ()  [unwired: 1 in, 5 out]
          n209 = case shown="True" "DB48" {
            frame False {
            }
            frame True {
              n210 = local write "Channels"("N4,N8,E4,E8,S4,S8,W4,W8" ("Channels")) -> ()
            }
          }
          n211 = case shown="True" "DB37" {
            frame False {
            }
            frame True {
              n212 = local write "Channels"("N3,N7,E3,E7,S3,S7,W3,W7" ("Channels")) -> ()
            }
          }
          n213 = case shown="True" "DB26" {
            frame False {
            }
            frame True {
              n214 = local write "Channels"("N2,N6,E2,E6,S2,S6,W2,W6" ("Channels")) -> ()
            }
          }
          n215 = case shown="True" "Device Banks" {
            frame False {
            }
            frame True {
              n216 = local write "Channels"("N1,N5,E1,E5,S1,S5,W1,W5" ("Channels")) -> ()
            }
          }
        }
        event "Record": Value Change {
          n217 = event-data() -> ()  [unwired: 1 in, 6 out]
          n218 = case shown="True" "Record" {
            tunnel: w312 -> [w314 w318]
            frame False {
              n219 = Enqueue Element(queue=w314, element=cluster{"Command":string} {"Command"="MonitorClose"}) -> (queue out=w316:refnum<queue>)  [unwired: 2 in, 2 out]
              n220 = Lossy Enqueue Element(queue=w316, element=cluster{"Command":string} {"Command"="File_Close"}) -> ()  [unwired: 1 in, 4 out]
            }
            frame True {
              n221 = local read "Recording"() -> (w319:bool)
              n222 = case shown="False" w319 {
                tunnel: w318 -> [w320 w322]
                frame False {
                  n223 = Lossy Enqueue Element(queue=w320, element=cluster{"Command":string} {"Command"="RT_Curve"}) -> ()  [unwired: 1 in, 4 out]
                }
                frame True {
                  n224 = Lossy Enqueue Element(queue=w322, element=cluster{"Command":string} {"Command"="FileClose"}) -> ()  [unwired: 1 in, 4 out]
                }
              }
            }
          }
        }
        event "IV Monitoring": Value Change {
          n225 = event-data() -> ()  [unwired: 1 in, 6 out]
          n226 = Enqueue Element(queue=w324, element=cluster{"Command":string} {"Command"="ParameterRead"}) -> (queue out=w325:refnum<queue>)  [unwired: 2 in, 2 out]
          n227 = Enqueue Element(queue=w325, element=cluster{"Command":string} {"Command"="MonitorOpen"}) -> (queue out=w327:refnum<queue>)  [unwired: 2 in, 2 out]
          n228 = Lossy Enqueue Element(queue=w327, element=cluster{"Command":string} {"Command"="IV_Curve"}) -> ()  [unwired: 1 in, 4 out]
        }
        event "Run Experiment": Value Change {
          n229 = event-data() -> ()  [unwired: 1 in, 6 out]
          n230 = Unbundle By Name(w332) -> ("ExperimentCommands"=w331:refnum<queue>)
          n231 = Enqueue Element(queue=w331, element=cluster{"Command":string} {"Command"="Run"}) -> ()  [unwired: 2 in, 3 out]
        }
        event "RT Monitoring": Value Change {
          n232 = event-data() -> ()  [unwired: 1 in, 6 out]
          n233 = local read "Monitoring"() -> (w335:bool)
          n234 = case shown="False" w335 {
            tunnel: w333 -> [w336 w339]
            frame False {
              n235 = Lossy Enqueue Element(queue=w336, element=cluster{"Command":string} {"Command"="MonitorOpen"}) -> ()  [unwired: 1 in, 4 out]
            }
            frame True {
              n236 = Lossy Enqueue Element(queue=w339, element=cluster{"Command":string} {"Command"="MonitorClose"}) -> ()  [unwired: 1 in, 4 out]
            }
          }
          "RT Monitoring 2" <- "RT Monitoring"
        }
        event "Clear Waste": Value Change {
          w342 = "air" ("analyte")
          n237 = event-data() -> ()  [unwired: 1 in, 6 out]
          n238 = local read "Pump"() -> (w352:refnum<k24>)
          n239 = local read "MaxSyringSpeed"() -> (w340:dbl)
          n240 = local read "SyringeVolume"() -> (w341:dbl)
          n241 = invoke class="Pump" method="Initalize"(reference=w352, "openAnalyte"="Air") -> (reference out=w350:refnum<k24>)  [unwired: 2 in, 3 out]
          n242 = for {
            N: 3 -> [_]
            tunnel: [w370] -> w351
            tunnel: w350 -> [w369]
            tunnel: [w363] -> w348
            tunnel: w340 -> [w362]
            tunnel: w341 -> [w361]
            tunnel: w342 -> [w360]
            n243 = invoke class="Pump" method="Pull"(reference=w369, "analyte"="Waste", "volume_uL"=w361, "speed_uL_s"=w362) -> (reference out=w367:refnum<k24>, "Pull"=w370:string)  [unwired: 2 in, 4 out]
            n244 = invoke class="Pump" method="Push"(reference=w367, "analyte"=w360, "volume_uL"=w361, "speed_uL_s"=w362) -> (reference out=w366:refnum<k24>)  [unwired: 2 in, 5 out]
            n245 = invoke class="Pump" method="Pull"(reference=w366, "analyte"="Water", "volume_uL"=w361, "speed_uL_s"=w362) -> (reference out=w364:refnum<k24>)  [unwired: 2 in, 5 out]
            n246 = invoke class="Pump" method="Push"(reference=w364, "analyte"=w360, "volume_uL"=w361, "speed_uL_s"=w362) -> (reference out=w363:refnum<k24>)  [unwired: 2 in, 5 out]
          }
          "Pull" <- w351
          n247 = for {
            N: 5 -> [_]
            tunnel: w348 -> [w359]
            tunnel: w341 -> [w356]
            tunnel: w340 -> [w355]
            tunnel: [w354] -> w345
            tunnel: w342 -> [w353]
            n248 = invoke class="Pump" method="Pull"(reference=w359, "analyte"="Dispense", "volume_uL"=w356, "speed_uL_s"=w355) -> (reference out=w357:refnum<k24>)  [unwired: 2 in, 5 out]
            n249 = invoke class="Pump" method="Push"(reference=w357, "analyte"=w353, "volume_uL"=w356, "speed_uL_s"=w355) -> (reference out=w354:refnum<k24>)  [unwired: 2 in, 5 out]
          }
          n250 = invoke class="Pump" method="Pull"(reference=w345, "analyte"="Waste", "volume_uL"=w341, "speed_uL_s"=w340) -> (reference out=w343:refnum<k24>)  [unwired: 2 in, 5 out]
          n251 = invoke class="Pump" method="Push"(reference=w343, "analyte"=w342, "volume_uL"=w341, "speed_uL_s"=w340) -> ()  [unwired: 2 in, 6 out]
        }
        event "ClearInput": Value Change {
          w376 = "Air" ("analyte")
          n252 = event-data() -> ()  [unwired: 1 in, 6 out]
          n253 = local read "Pump"() -> (w378:refnum<k24>)
          n254 = invoke class="Pump" method="Initalize"(reference=w378, "openAnalyte"="air") -> (reference out=w374:refnum<k24>)  [unwired: 2 in, 3 out]
          n255 = local read "MaxSyringSpeed"() -> (w371:dbl)
          n256 = local read "SyringeVolume"() -> (w372:dbl)
          n257 = for {
            N: 3 -> [_]
            tunnel: w374 -> [w386]
            tunnel: w372 -> [w383]
            tunnel: w371 -> [w382]
            tunnel: [w381] -> w377
            tunnel: w376 -> [w380]
            n258 = invoke class="Pump" method="Pull"(reference=w386, "analyte"="Waste", "volume_uL"=w383, "speed_uL_s"=w382) -> (reference out=w384:refnum<k24>)  [unwired: 2 in, 5 out]
            n259 = invoke class="Pump" method="Push"(reference=w384, "analyte"=w380, "volume_uL"=w383, "speed_uL_s"=w382) -> (reference out=w381:refnum<k24>)  [unwired: 2 in, 5 out]
          }
          n260 = for {
            N: 4 -> [_]
            tunnel: w377 -> [w393]
            tunnel: w372 -> [w390]
            tunnel: w371 -> [w389]
            tunnel: [w388] -> _
            tunnel: w376 -> [w387]
            n261 = invoke class="Pump" method="Pull"(reference=w393, "analyte"="Dispense", "volume_uL"=w390, "speed_uL_s"=w389) -> (reference out=w391:refnum<k24>)  [unwired: 2 in, 5 out]
            n262 = invoke class="Pump" method="Push"(reference=w391, "analyte"=w387, "volume_uL"=w390, "speed_uL_s"=w389) -> (reference out=w388:refnum<k24>)  [unwired: 2 in, 5 out]
          }
        }
        event "CleanAll": Value Change {
          w396 = 10
          n263 = event-data() -> ()  [unwired: 1 in, 6 out]
          n264 = local read "MaxSyringSpeed"() -> (w394:dbl)
          n265 = local read "SyringeVolume"() -> (w395:dbl)
          n266 = local read "Pump"() -> (w399:refnum<k24>)
          n267 = for {
            N: w396 -> [_]
            tunnel: w399 -> [w419]
            tunnel: w395 -> [w415]
            tunnel: w394 -> [w414]
            tunnel: [w413] -> w398
            n268 = invoke class="Pump" method="Pull"(reference=w419, "analyte"="water", "volume_uL"=w415, "speed_uL_s"=w414) -> (reference out=w417:refnum<k24>)  [unwired: 2 in, 5 out]
            n269 = invoke class="Pump" method="Push"(reference=w417, "analyte"="MPA", "volume_uL"=w415, "speed_uL_s"=w414) -> (reference out=w413:refnum<k24>)  [unwired: 2 in, 5 out]
          }
          n270 = for {
            N: w396 -> [_]
            tunnel: w398 -> [w412]
            tunnel: w395 -> [w408]
            tunnel: w394 -> [w407]
            tunnel: [w406] -> w397
            n271 = invoke class="Pump" method="Pull"(reference=w412, "analyte"="water", "volume_uL"=w408, "speed_uL_s"=w407) -> (reference out=w410:refnum<k24>)  [unwired: 2 in, 5 out]
            n272 = invoke class="Pump" method="Push"(reference=w410, "analyte"="Dispense", "volume_uL"=w408, "speed_uL_s"=w407) -> (reference out=w406:refnum<k24>)  [unwired: 2 in, 5 out]
          }
          n273 = for {
            N: w396 -> [_]
            tunnel: w397 -> [w405]
            tunnel: w395 -> [w401]
            tunnel: w394 -> [w400]
            n274 = invoke class="Pump" method="Pull"(reference=w405, "analyte"="water", "volume_uL"=w401, "speed_uL_s"=w400) -> (reference out=w403:refnum<k24>)  [unwired: 2 in, 5 out]
            n275 = invoke class="Pump" method="Push"(reference=w403, "analyte"="TimEtch", "volume_uL"=w401, "speed_uL_s"=w400) -> ()  [unwired: 2 in, 6 out]
          }
        }
        event "TimeEtch Back": Value Change {
          n276 = event-data() -> ()  [unwired: 1 in, 6 out]
          n277 = local read "MaxSyringSpeed"() -> (w420:dbl)
          n278 = local read "SyringeVolume"() -> (w421:dbl)
          n279 = local read "Pump"() -> (w424:refnum<k24>)
          n280 = for {
            N: 3 -> [_]
            tunnel: w424 -> [w431]
            tunnel: w421 -> [w428]
            tunnel: w420 -> [w427]
            tunnel: [w426] -> _
            tunnel: "air" ("analyte") -> [w425]
            n281 = invoke class="Pump" method="Pull"(reference=w431, "analyte"="Timetch", "volume_uL"=w428, "speed_uL_s"=w427) -> (reference out=w429:refnum<k24>)  [unwired: 2 in, 5 out]
            n282 = invoke class="Pump" method="Push"(reference=w429, "analyte"=w425, "volume_uL"=w428, "speed_uL_s"=w427) -> (reference out=w426:refnum<k24>)  [unwired: 2 in, 5 out]
          }
        }
        event "MPA Load": Value Change {
          w434 = 100.0 ("speed_uL_s")
          w433 = "MPA" ("analyte")
          n283 = event-data() -> ()  [unwired: 1 in, 6 out]
          n284 = local read "Pump"() -> (w442:refnum<k24>)
          n285 = invoke class="Pump" method="Initalize"(reference=w442, "openAnalyte"="air") -> (reference out=w441:refnum<k24>)  [unwired: 2 in, 3 out]
          n286 = local read "SyringeVolume"() -> (w432:dbl)
          n287 = invoke class="Pump" method="Pull"(reference=w441, "analyte"="dispense", "volume_uL"=w432, "speed_uL_s"=w434) -> (reference out=w439:refnum<k24>)  [unwired: 2 in, 5 out]
          n288 = invoke class="Pump" method="Push"(reference=w439, "analyte"=w433, "volume_uL"=w432, "speed_uL_s"=w434) -> (reference out=w435:refnum<k24>)  [unwired: 2 in, 5 out]
          n289 = invoke class="Pump" method="Pull"(reference=w435, "analyte"="dispense", "volume_uL"=w432, "speed_uL_s"=w434) -> (reference out=w437:refnum<k24>)  [unwired: 2 in, 5 out]
          n290 = invoke class="Pump" method="Push"(reference=w437, "analyte"=w433, "volume_uL"=w432, "speed_uL_s"=w434) -> ()  [unwired: 2 in, 6 out]
        }
        event "CleanPort": Value Change {
          n291 = event-data() -> ()  [unwired: 1 in, 6 out]
          n292 = local read "MaxSyringSpeed"() -> (w445:dbl)
          n293 = local read "SyringeVolume"() -> (w444:dbl)
          n294 = local read "Pump"() -> (w450:refnum<k24>)
          n295 = for {
            N: 5 -> [_]
            tunnel: w450 -> [w457]
            tunnel: w444 -> [w454]
            tunnel: w445 -> [w453]
            tunnel: [w452] -> w447
            tunnel: "Port To Clean" -> [w451]
            n296 = invoke class="Pump" method="Pull"(reference=w457, "analyte"="Water", "volume_uL"=w454, "speed_uL_s"=w453) -> (reference out=w455:refnum<k24>)  [unwired: 2 in, 5 out]
            n297 = invoke class="Pump" method="Push"(reference=w455, "analyte"=w451, "volume_uL"=w454, "speed_uL_s"=w453) -> (reference out=w452:refnum<k24>)  [unwired: 2 in, 5 out]
          }
          n298 = invoke class="Pump" method="Pull"(reference=w447, "analyte"="Air", "volume_uL"=w444, "speed_uL_s"=w445) -> (reference out=w448:refnum<k24>)  [unwired: 2 in, 5 out]
          n299 = invoke class="Pump" method="Push"(reference=w448, "analyte"="Port To Clean", "volume_uL"=w444, "speed_uL_s"=w445) -> ()  [unwired: 2 in, 6 out]
        }
        event "LoadPort": Value Change {
          n300 = event-data() -> ()  [unwired: 1 in, 6 out]
          n301 = local read "Port To Clean"() -> (w466:string)
          n302 = local read "SyringeVolume"() -> (w459:dbl)
          n303 = local read "MaxSyringSpeed"() -> (w458:dbl)
          n304 = local read "Pump"() -> (w467:refnum<k24>)
          n305 = invoke class="Pump" method="Pull"(reference=w467, "analyte"=w466, "volume_uL"=w459, "speed_uL_s"=w458) -> (reference out=w464:refnum<k24>)  [unwired: 2 in, 5 out]
          n306 = for {
            N: 2 -> [_]
            tunnel: w464 -> [w474]
            tunnel: w459 -> [w470]
            tunnel: w458 -> [w469]
            tunnel: [w468] -> w460
            n307 = invoke class="Pump" method="Pull"(reference=w474, "analyte"="water", "volume_uL"=w470, "speed_uL_s"=w469) -> (reference out=w472:refnum<k24>)  [unwired: 2 in, 5 out]
            n308 = invoke class="Pump" method="Push"(reference=w472, "analyte"="air", "volume_uL"=w470, "speed_uL_s"=w469) -> (reference out=w468:refnum<k24>)  [unwired: 2 in, 5 out]
          }
          n309 = invoke class="Pump" method="Pull"(reference=w460, "analyte"="waste", "volume_uL"=w459, "speed_uL_s"=w458) -> (reference out=w462:refnum<k24>)  [unwired: 2 in, 5 out]
          n310 = invoke class="Pump" method="Push"(reference=w462, "analyte"="air", "volume_uL"=w459, "speed_uL_s"=w458) -> ()  [unwired: 2 in, 6 out]
        }
        event "PrimeWater": Value Change {
          n311 = event-data() -> ()  [unwired: 1 in, 6 out]
          n312 = local read "MaxSyringSpeed"() -> (w475:dbl)
          n313 = local read "SyringeVolume"() -> (w476:dbl)
          n314 = local read "Pump"() -> (w480:refnum<k24>)
          n315 = for {
            N: 3 -> [_]
            tunnel: w480 -> [w493]
            tunnel: [w489] -> w478
            tunnel: w476 -> [w488]
            tunnel: w475 -> [w487]
            n316 = invoke class="Pump" method="Pull"(reference=w493, "analyte"="water", "volume_uL"=w488, "speed_uL_s"=w487) -> (reference out=w491:refnum<k24>)  [unwired: 2 in, 5 out]
            n317 = invoke class="Pump" method="Push"(reference=w491, "analyte"="air", "volume_uL"=w488, "speed_uL_s"=w487) -> (reference out=w489:refnum<k24>)  [unwired: 2 in, 5 out]
          }
          n318 = for {
            N: 3 -> [_]
            tunnel: w478 -> [w486]
            tunnel: w476 -> [w482]
            tunnel: w475 -> [w481]
            n319 = invoke class="Pump" method="Pull"(reference=w486, "analyte"="waste", "volume_uL"=w482, "speed_uL_s"=w481) -> (reference out=w484:refnum<k24>)  [unwired: 2 in, 5 out]
            n320 = invoke class="Pump" method="Push"(reference=w484, "analyte"="air", "volume_uL"=w482, "speed_uL_s"=w481) -> ()  [unwired: 2 in, 6 out]
          }
        }
        event "Wafer, Chip", "Experiment Name", "Bias Voltage (mV)", "Reference Voltage (mV)", "Notes", "Buffer", "Analyte": Value Change {
          n321 = event-data() -> ()  [unwired: 1 in, 6 out]
          n322 = Enqueue Element(queue=w494, element=cluster{"Command":string} {"Command"="ParameterRead"}) -> ()  [unwired: 2 in, 3 out]
        }
      }
      n323 = local read "StopProgram"() -> (w303:bool)
    }
  }
  n324 = while "Display Loop" {
    tunnel: w2 -> [_]
    tunnel: w1 -> [w517]
    stop <- w519 stop-if-true
    n325 = Unbundle By Name(w517) -> ("DisplayCurrents"=w518:refnum<queue>)
    n326 = Flush Queue(queue=w518) -> (remaining elements=w516:cluster{waveform(dbl)[]}[])  [unwired: 1 in, 2 out]
    n327 = Array Size(array=w516) -> (size(s)=w514:i32)
    n328 = Greater Than 0?(x=w514) -> (x > 0?=w515:bool)
    n329 = case shown="True" w515 {
      tunnel: w517 -> [_ w530]
      tunnel: w516 -> [_ w529]
      tunnel: w514 -> [_ _]
      frame False {
      }
      frame True {
        (unwired) 0 ("index")
        n330 = Index Array(array=w529) -> (element=w528:cluster{waveform(dbl)[]})  [unwired: 1 in]
        n331 = Unbundle(w528) -> (w523:waveform(dbl)[])
        n332 = local read "MeasureMode"() -> (w539:enum32{"RT Monitor", "IV Monitor"})
        n333 = local read "Monitoring"() -> (w546:bool)
        n334 = property on="Tab Control 2" class="TabCtl (strict)"() -> ("Value"=w547:T2)  [unwired: 2 in, 2 out]
        n335 = Array Size(array=w523) -> (size(s)=w521:i32)
        n336 = for {
          tunnel: w547 -> [w556]
          tunnel: w546 -> [w555]
          tunnel: w539 -> [w554]
          tunnel: w530 -> [_]
          tunnel: w529 -> [w553] mode=indexing
          n337 = Unbundle(w553) -> (w550:waveform(dbl)[])
          n338 = Array Size(array=w550) -> (size(s)=w551:i32)
          n339 = Decrement(x=w551) -> (x-1=w548:i32)
          n340 = Index Array(array=w550, index=w548) -> (element=w552:waveform(dbl))
          n341 = Array Subset(array=w550, length=w548) -> (w549:waveform(dbl)[])  [unwired: 1 in]
          n342 = case shown="True" w555 {
            tunnel: w556 -> [_ w560]
            tunnel: w552 -> [_ w559]
            tunnel: w549 -> [_ w558]
            tunnel: w554 -> [_ w557]
            frame False {
            }
            frame True {
              n343 = case shown="\"View All\"" w560 {
                tunnel: w558 -> [w565 w568 w569]
                tunnel: w559 -> [_ w567 w574]
                tunnel: w557 -> [_ w566 _]
                frame "RT Monitor", Default {
                  n344 = call "SortRTTraces.vi"("Array in"=w565) -> ("Array 7"=→"Channel 3":waveform(dbl)[], "Array 5"=→"Channel 2":waveform(dbl)[], "Array 6"=→"Channel 1":waveform(dbl)[], "Array 4"=→"Channel 4":waveform(dbl)[])  [unwired: 7 in]
                }
                frame "View All" {
                  n345 = call "ShowAll.vi"("Tab Control 2"=w566, "Bias"=w567, "Traces"=w568) -> ()  [unwired: 9 in]
                }
                frame "IV Monitor" {
                  n346 = call "SortIVTraces.vi"("Array in"=w569, "Waveform"=w574) -> ("Array 6"=→"XY Graph 3":cluster{"Y":dbl[], "Y":dbl[]}[], "Array 3"=→"XY Graph 4":cluster{"Y":dbl[], "Y":dbl[]}[], "Array 4"=→"XY Graph 2":cluster{"Y":dbl[], "Y":dbl[]}[], "Array 5"=→"XY Graph":cluster{"Y":dbl[], "Y":dbl[]}[])  [unwired: 5 in, 1 out]
                }
              }
            }
          }
        }
        n347 = Decrement(x=w521) -> (x-1=w520:i32)
        n348 = Array Subset(array=w523, length=w520) -> (w522:waveform(dbl)[])  [unwired: 1 in]
        n349 = local read "Bias Voltage (mV)"() -> (w538:string)
        n350 = case shown="\"RT Monitor\", Default" w539 {
          tunnel: w522 -> [w577 w584]
          tunnel: [w576 w582] -> w537
          tunnel: [w575 w583] -> w536
          frame "RT Monitor", Default {
            n351 = for {
              tunnel: w577 -> [w581] mode=indexing
              tunnel: [w578] -> w576 mode=indexing
              tunnel: [w580] -> w575 mode=indexing
              n352 = call <vilib>:"Waveform Min Max.vi"("waveform in"=w581) -> ("Y min"=w579:dbl, "Y max"=w580:dbl)  [unwired: 5 in, 4 out]
              n353 = Subtract(x=w580, y=w579) -> (x-y=w578:dbl)
            }
          }
          frame "IV Monitor" {
            n354 = for {
              tunnel: w584 -> [w587] mode=indexing
              tunnel: [w585] -> w583 mode=indexing
              tunnel: [0.0] -> w582 mode=indexing
              n355 = call <vilib>:"Waveform Min Max.vi"("waveform in"=w587) -> ("Y max"=w585:dbl)  [unwired: 5 in, 5 out]
            }
          }
        }
        n356 = Decimal String To Number(string=w538) -> (number=w525:i32)  [unwired: 2 in, 1 out]
        n357 = Divide(x=w525, y=1000) -> (x/y=w526:dbl)
        n358 = local read "LastPoint"() -> (w544:i64)
        n359 = Get Date/Time In Seconds() -> (seconds since 1Jan1904=w545:timestamp)
        n360 = Add(x=w526, y=0.001) -> (x+y=w532:dbl)
        n361 = To Quad Integer(1:w545) -> (0:w540:i64)
        n362 = Add(x=w544, y=i64 15) -> (x+y=w542:i64)
        n363 = local read "ChannelHistory"() -> (w533:refnum<k24>)
        n364 = Greater?(x=w540, y=w542) -> (0:w541:bool)
        n365 = Divide(x=w536, y=w532) -> (x/y=w534:dbl[])
        n366 = Divide(x=w537, y=w532) -> (x/y=w535:dbl[])
        n367 = case shown="True" w541 {
          tunnel: w540 -> [_ w613]
          tunnel: w533 -> [_ w612]
          frame False {
          }
          frame True {
            n368 = invoke class="ChannelDictionary" method="DataPoint"(reference=w612) -> (reference out=w611:refnum<k24>)  [unwired: 2 in, 2 out]
            n369 = invoke class="ChannelDictionary" method="ChannelNames"(reference=w611) -> (reference out=w609:refnum<k24>, "ChannelNames"=w610:string[])  [unwired: 2 in, 1 out]
            n370 = invoke class="ChannelDictionary" method="GetTimes"(reference=w609) -> ("GetTimes"=w608:dbl[])  [unwired: 2 in, 2 out]
            n371 = for {
              tunnel: w610 -> [w619] mode=indexing
              tunnel: w609 -> [w622]
              tunnel: w608 -> [w621]
              tunnel: [w620] -> w607 mode=indexing
              tunnel: [w614] -> w606 mode=indexing
              n372 = invoke class="ChannelDictionary" method="GetChannel"(reference=w622, "channel"=w619) -> ("GetChannel"=w618:dbl[])  [unwired: 2 in, 3 out]
              n373 = Bundle("GetTimes"=w621, "GetChannel"=w618) -> (w620:cluster{"GetTimes":dbl[], "GetChannel":dbl[]})  [unwired: 1 in]
              n374 = call-poly <vilib>:"Mean.vi"("X"=w618) -> ("mean"=w617:dbl)  [unwired: 1 out]
              n375 = Number To Fractional String(number=w617) -> (F-format string=w616:string)  [unwired: 3 in]
              n376 = Build Array(w619, w616, "" ("element")) -> (w614:string[])
            }
            "History" <- w607
            "Stats" <- w606
            "LastPoint" <- w613
          }
        }
        n377 = for {
          tunnel: w533 -> [w588]
          tunnel: w522 -> [w596] mode=indexing
          tunnel: w534 -> [w595] mode=indexing
          tunnel: w535 -> [w594] mode=indexing
          tunnel: [w593] -> w527 mode=indexing
          n378 = Absolute Value(x=w595) -> (abs(x)=w592:dbl)
          n379 = Get Waveform Attribute(6:"NI_ChannelName" ("name"), 7:w596) -> (1:w598:variant)  [unwired: 2 in, 3 out]
          n380 = Variant To Data(type="", Variant=w598) -> (data=w591:string)  [unwired: 1 in, 1 out]
          n381 = Not Equal?(x=w591, y="Bias") -> (x != y?=w589:bool)
          n382 = case shown="True" w589 {
            tunnel: w588 -> [_ w605]
            tunnel: w594 -> [_ w604]
            tunnel: [0.0 ("AddAverage7") w603] -> w593
            tunnel: w592 -> [_ w602]
            tunnel: w591 -> [_ w601]
            frame False {
            }
            frame True {
              n383 = invoke class="ChannelDictionary" method="AddAverage7"(reference=w605, "channel"=w601, "mean"=w602, "std"=w604) -> ("AddAverage7"=w603:dbl)  [unwired: 2 in, 5 out]
            }
          }
        }
        "Array" <- w527
      }
    }
    n384 = local read "StopProgram"() -> (w519:bool)
  }
  n385 = while {
    tunnel: w1 -> [w626]
    stop <- w625 stop-if-true
    n386 = Unbundle By Name(w626) -> ("MonitorCurrents"=w628:refnum<queue>)
    n387 = Flush Queue(queue=w628) -> (remaining elements=w627:T7)  [unwired: 1 in, 2 out]
    n388 = local read "MeasureMode"() -> (w629:enum32{"RT Monitor", "IV Monitor"})
    n389 = local read "tdms file out"() -> (w623:refnum<k34>)
    n390 = for {
      tunnel: w629 -> [w635]
      tunnel: w627 -> [w634] mode=indexing
      shift-right: [w631] -> w624
      shift-left: w623 -> [w630]
      n391 = Unbundle(w634) -> ("Waveforms"=w633:waveform(dbl)[])  [unwired: 1 out]
      n392 = case shown="True" TRUE ("FileOpen") {
        tunnel: w633 -> [_ w645]
        tunnel: w635 -> [_ _]
        tunnel: w630 -> [w636 w638]
        tunnel: [w636 w637] -> w631
        frame False {
        }
        frame True {
          n393 = local read "ParameterNames"() -> (w641:string[])
          n394 = local read "ParameterValues"() -> (w640:string[])
          n395 = local read "fileCreateTime"() -> (w643:timestamp)
          n396 = local read "output path"() -> (w642:path)
          n397 = local read "Analyte"() -> (w639:string)
          n398 = call "SaveFiles.vi"("Refnum in"=w638, "Analyte"=w639, "fileCreateTime"=w643, "Array 2"=w645, "ParameterValues"=w640, "output path"=w642, "ParameterNames"=w641) -> ("Refnum out"=w637:refnum<k34>, "seconds since 1Jan1904"=w644:timestamp)  [unwired: 11 in]
          n399 = local write "fileCreateTime"(w644) -> ()
        }
      }
    }
    n400 = local write "tdms file out"(w624) -> ()
    n401 = local read "StopProgram"() -> (w625:bool)
  }
  n402 = while {
    tunnel: w1 -> [w647]
    tunnel: w3 -> [w649]
    stop <- w646 stop-if-true
    n403 = Unbundle By Name(w647) -> ("ExperimentCommands"=w648:refnum<queue>)
    n404 = Dequeue Element(queue=w648) -> (element=w650:cluster{"Command":string})  [unwired: 2 in, 3 out]
    n405 = flat-sequence {
      tunnel: w650 -> [w660]
      tunnel: w649 -> [w658]
      tunnel: w647 -> [w657]
      frame #0 {
        n406 = Unbundle By Name(w660) -> ("Command"=w659:string)
        n407 = local read "Running Experiment"() -> (w652:bool)
        n408 = control-ref of="Bias Voltage (mV)"() -> (w656:refnum<vi>)
        n409 = local read "Experiment"() -> (w653:string[][])
        n410 = control-ref of="Current Step"() -> (w651:refnum<vi>)
        n411 = control-ref of="TraceTime"() -> (w655:refnum<vi>)
        n412 = control-ref of="Analyte"() -> (w654:refnum<vi>)
        n413 = case shown="\"Run\"" w659 {
          tunnel: w658 -> [_ w669 _]
          tunnel: w657 -> [_ w668 _]
          tunnel: w656 -> [_ w667 _]
          tunnel: w655 -> [_ w666 _]
          tunnel: w654 -> [_ w665 _]
          tunnel: w653 -> [_ w664 _]
          tunnel: w652 -> [_ _ _]
          tunnel: w651 -> [_ w663 _]
          frame "False", Default {
          }
          frame "Run" {
            n414 = flat-sequence {
              tunnel: w664 -> [w677]
              tunnel: [w677] -> w662
              tunnel: [w670] -> w661
              tunnel: w669 -> [w687]
              tunnel: w668 -> [w686]
              tunnel: w667 -> [w685]
              tunnel: w666 -> [w684]
              tunnel: w665 -> [w683]
              tunnel: w663 -> [w681]
              tunnel: w662 -> [w682]
              tunnel: w661 -> [w680]
              frame #0 {
                n415 = local read "Reference Voltage (mV)"() -> (w674:string)
                n416 = local read "Experiment Name"() -> (w676:string)
                n417 = local read "Wafer, Chip"() -> (w675:string)
                n418 = Empty String/Path?(string/path=w676) -> (empty?=w673:bool)
                n419 = Empty String/Path?(string/path=w675) -> (empty?=w672:bool)
                n420 = Empty String/Path?(string/path=w674) -> (empty?=w671:bool)
                n421 = Compound Arithmetic op=OR(w673, w672, w671) -> (w670:bool)
                n422 = case shown="True" w670 {
                  frame False {
                  }
                  frame True {
                    n423 = One Button Dialog(message="Please set experiment name, Wafer/Chip, and reference electrodes") -> ()  [unwired: 1 in, 1 out]
                  }
                }
              }
              frame #1 {
                n424 = case shown="False" w680 {
                  tunnel: w687 -> [w699 _]
                  tunnel: w686 -> [w696 _]
                  tunnel: w685 -> [w695 _]
                  tunnel: w684 -> [w694 _]
                  tunnel: w683 -> [w693 _]
                  tunnel: w682 -> [w692 _]
                  tunnel: w681 -> [w691 _]
                  frame False {
                    n425 = invoke class="Pump" method="Initalize"(reference=w699, "openAnalyte"="AIR") -> (reference out=w697:refnum<k24>)  [unwired: 2 in, 3 out]
                    n426 = Get Date/Time In Seconds() -> (seconds since 1Jan1904=w690:timestamp)
                    n427 = local read "SyringeVolume"() -> (w688:dbl)
                    n428 = To Quad Integer(1:w690) -> (0:w689:i64)
                    n429 = local write "First Time"(w689) -> ()
                    n430 = call "RunStep.vi"("syringe_volume_uL"=w688, "MessageQueues"=w696, "Experiment"=w692, "Current Step 2"=w691, "Pump Class"=w697, "Bias"=w695, "TimeTrace"=w694, "Analyte"=w693) -> ()  [unwired: 4 in]
                    "Running Experiment" <- TRUE ("Running Experiment")
                  }
                  frame True {
                  }
                }
                n431 = local read "ChannelHistory"() -> (w679:refnum<k24>)
                n432 = invoke class="ChannelDictionary" method="Restart"(reference=w679) -> ()  [unwired: 2 in, 3 out]
              }
            }
          }
          frame "Step" {
          }
        }
      }
    }
    n433 = local read "StopProgram"() -> (w646:bool)
  }
